vi "generate file error.vi"(4 "message":string, 5 "call chain?":bool, 6 "source":string, 7 "severity":T1=enum."operation failed", 8 "exception in":T2 {"code" format="%.0x"}, 10 "file path":path, 11 "file error":T4) -> (0 "exception":T2 {"code" format="%.0x"})   [LabVIEW 2013, in "file errors.lvlib"]
uses:
  file errors.lvlib
  file error.ctl
  exception.ctl
  context.ctl
  severity.ctl
  Variant Repository/Write Variant Repository/Write Exception Property.xnode
  exception.lvlib
  <vilib>/Utility/VariantDataType/GetTypeInfo.vi
  <vilib>/Utility/VariantDataType/VariantType.lvlib
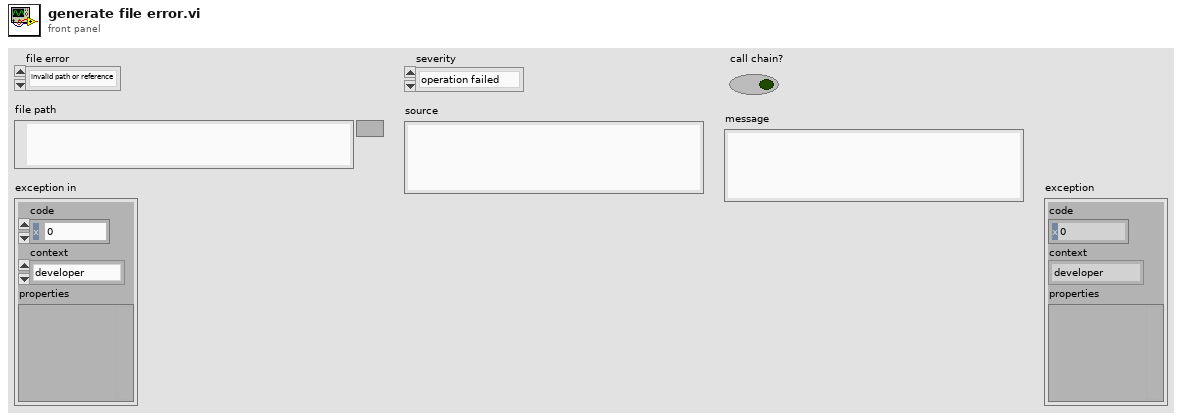
[diagram p1: front panel]
types:
  T1 = typedef "exception.lvlib/severity.ctl" = enum8{"unspecified", "informational", "operation failed", "data corruption", "system corruption", "critical unknown state"}
  T2 = typedef "exception.lvlib/exception.ctl" = cluster{"code":i32, "context":T3, "properties":variant}
  T3 = typedef "exception.lvlib/context.ctl" = enum16{"developer", "user interface", "standard", "limited", "deterministic"}
  T4 = typedef "file errors.lvlib/file error.ctl" = enum16{"invalid path or reference", "end of file", "file already opened", "generic file error", "file not found", "permissions invalid", "disk full", "duplicate path", "too many open file handles", "useless generic error"}
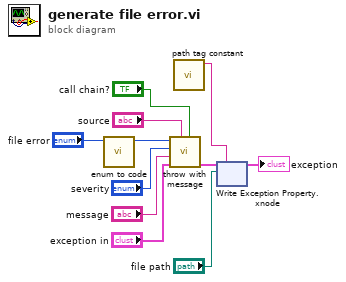
[diagram p0: block diagram]
diagram:
  n1 = call "enum to code.vi"("file error"="file error") -> ("code"=w1:i32)  [unwired: 10 in]
  n2 = call "throw with message.vi"("call chain?"="call chain?", "source"="source", "exception in"="exception in", "message"="message", "severity"="severity", "code"=w1) -> ("exception out"=w6:T2)  [unwired: 5 in]
  n3 = call "path tag constant.vi"() -> ("Tag"=w3:string)  [unwired: 11 in]
  n4 = xnode "Write Exception Property.xnode"("exception in"=w6, "Tag"=w3, "Value"="file path") -> ("exception out"=→"exception":T2)  [unwired: 1 out]
